vi "Parse State Queue Performance Test.vi"() -> ()   [LabVIEW 2020]
panel:
  out "Times Faster":dbl format="%#.2g"
  out "Waveform Chart":u32(graph)
  out "New":u32
  out "Old":u32
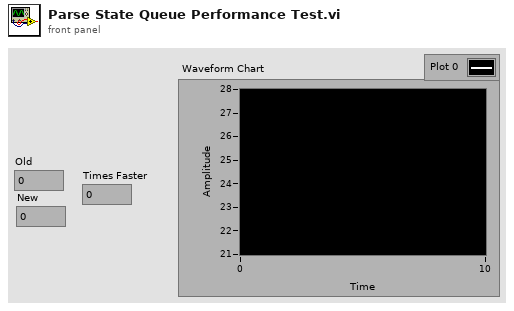
[diagram p1: front panel]
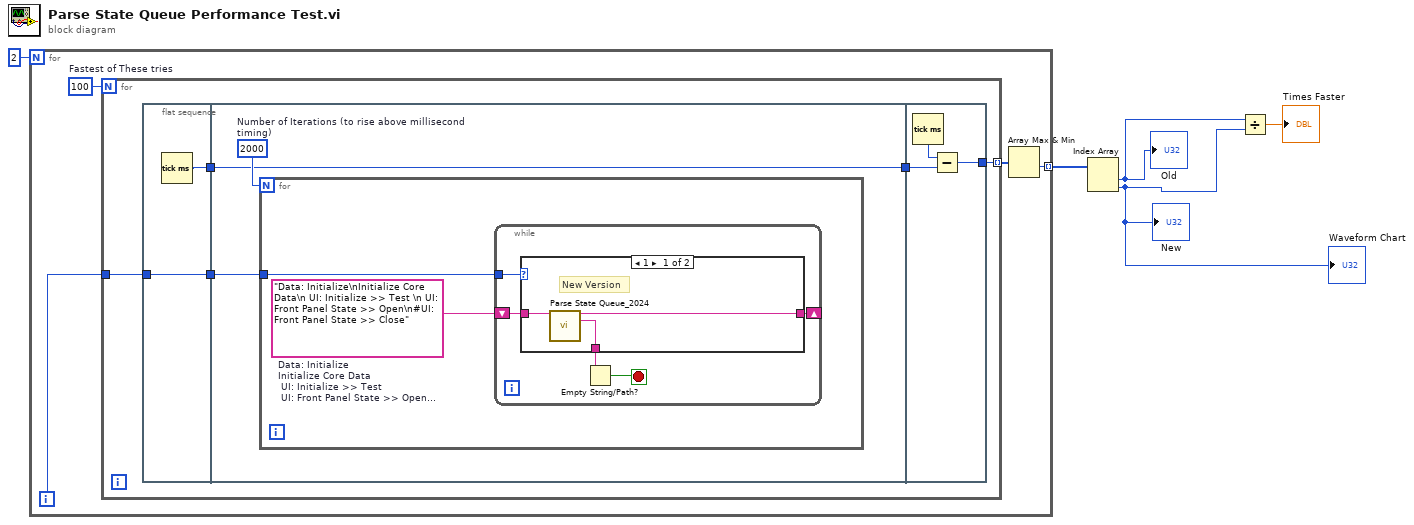
[diagram p0: block diagram]
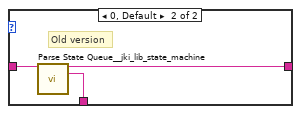
[diagram p2: hidden frame]
diagram:
  n1 = for {
    N: 2 -> [_]
    tunnel: [w6] -> w4 mode=indexing
    i -> [w9]
    w7 = 100  # Fastest of These tries
    n2 = for {
      N: w7 -> [_]
      tunnel: w9 -> [w11]
      tunnel: [w10] -> w8 mode=indexing
      n3 = flat-sequence {
        tunnel: [w16] -> w14
        tunnel: w11 -> [w15]
        tunnel: [w15] -> w13
        tunnel: w14 -> [w18]
        tunnel: [w18] -> w12
        tunnel: w13 -> [w17]
        tunnel: w12 -> [w34]
        tunnel: [w33] -> w10
        frame #0 {
          n4 = Tick Count (ms)() -> (millisecond timer value=w16:u32)
        }
        frame #1 {
          w19 = 2000  # Number of Iterations (to rise above millisecond timing)
          n5 = for {
            N: w19 -> [_]
            tunnel: w17 -> [w20]
            w21 = "Data: Initialize\nInitialize Core Data\n UI: Initialize >> Test \n UI: Front Panel State >> Open\n#UI: Front Panel State >> Close"  # Data: Initialize Initialize Core Data  UI: Initialize >> Test   UI: Front Panel State >> Open #UI: Front Panel State >> Close
            n6 = while {
              shift-right: [w23] -> _
              shift-left: w21 -> [w26]
              tunnel: w20 -> [w22]
              stop <- w24 stop-if-true
              n7 = case shown="1" w22 {
                tunnel: w26 -> [w29 w32]
                tunnel: [w28 w31] -> w25
                tunnel: [w27 w30] -> w23
                frame 1 {
                  # "New Version"
                  n8 = call "Parse State Queue_2024.vi"("State Queue"=w29) -> ("Remaining States"=w27:string, "Current State"=w28:string)  [unwired: 12 in, 1 out]
                }
                frame 0, Default {
                  # "Old version"
                  n9 = call <vilib>:"Parse State Queue__jki_lib_state_machine.vi"("State Queue"=w32) -> ("Remaining States"=w30:string, "Current State"=w31:string)  [unwired: 12 in, 1 out]
                }
              }
              n10 = Empty String/Path?(string/path=w25) -> (empty?=w24:bool)
            }
          }
        }
        frame #2 {
          n11 = Tick Count (ms)() -> (millisecond timer value=w35:u32)
          n12 = Subtract(x=w35, y=w34) -> (x-y=w33:u32)
        }
      }
    }
    n13 = Array Max & Min(array=w8) -> (min value=w6:u32)  [unwired: 3 out]
  }
  n14 = Index Array(array=w4) -> (element #1=w2:u32, element #2=w1:u32)  [unwired: 2 in]
  "Old" <- w2
  "New" <- w1
  "Waveform Chart" <- w1
  n15 = Divide(x=w2, y=w1) -> (x/y=→"Times Faster":dbl)
